vi "InitPneumatic.vi"   [LabVIEW 2015]
uses:
  <vilib>/Rock Robotics/WPI/Utilities/WPI_GetSetVariantRefNum.vi
types:
  T1 = typedef "constants.ctl" = cluster{"motorConstants":cluster{"leftDriveMotor":u8, "rightDriveMotor":u8, "climberAngler":i32, "climberWinch":T2, "shooterTopFlyWheel":T2, "shooterBottomFlyWheel":T2, "climberExtender":i32, "shooterIntakeWheel":T2}, "arduinoInputChannel":cluster{"armAngleUp":i32, "intakeWheelSpinIn":i32, "winchUp":i32, "extenderUp":i32, "AimingAuto":i32, "extenderDown":i32, "FrontArmAxis":i32}, "driveConstants":cluster{"firstIntervalPercent":dbl, "secondIntervalPercent":dbl, "thirdIntervalPercent":dbl}, "cRioInputChanels":cluster{"photoEye":i32, "limitExtender":i32}, "pneumaticsChannels":cluster{"angleSolenoid":T3, "shooterAnglerPneumaticForward":T3, "shooterAnglerPneumaticReverse":T3, "Pneumatics Control Module":u8}, "flyWheelConstants":cluster{"manualTopWheel":dbl, "manualBottomWheel":dbl, "autoFuncConst1":dbl, "autoFuncConst2":dbl, "autoFuncConst3":dbl, "autoFuncConst4":dbl, "Array":dbl[][]}, "Front Arm":cluster{"Arm Motor":u8}}
  T2 = typedef "FPGA_DIOPWMChannel.ctl" = enum8{"PWM 0", "PWM 1", "PWM 2", "PWM 3", "PWM 4", "PWM 5", "PWM 6", "PWM 7", "PWM 8", "PWM 9", "PWM MXP 0", "PWM MXP 1", "PWM MXP 2", "PWM MXP 3", "PWM MXP 4", "PWM MXP 5", "PWM MXP 6", "PWM MXP 7", "PWM MXP 8", "PWM MXP 9", "Invalid"}
  T3 = typedef "WPI_SolenoidChannel.ctl" = enum8{"Solenoid 0", "Solenoid 1", "Solenoid 2", "Solenoid 3", "Solenoid 4", "Solenoid 5", "Solenoid 6", "Solenoid 7", "Invalid"}
  T4 = typedef "WPI_CompressorDevRef.ctl" = cluster{"DevStatus":errorcluster, "Pneumatics Control Module":u8}
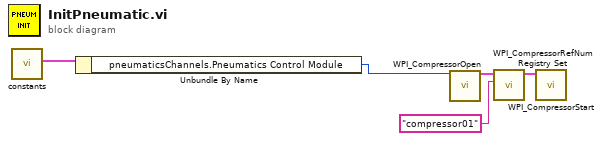
[diagram p0: block diagram]
diagram:
  n1 = call "constants.vi"() -> (2:w2:T1)  [unwired: 11 in]
  n2 = Unbundle By Name(w2) -> ("pneumaticsChannels.Pneumatics Control Module"=w1:u8)
  n3 = call <vilib>:"WPI_CompressorOpen.vi"("Pneumatics Control Module (0)"=w1) -> ("CompressorDevRef"=w3:T4)  [unwired: 13 in, 1 out]
  n4 = call <vilib>:"WPI_CompressorRefNum Registry Set.vi"("refnum name"="compressor01", "CompressorDevRef"=w3) -> ("CompressorDevRef"=w5:T4)  [unwired: 8 in, 1 out]
  n5 = call <vilib>:"WPI_CompressorStart.vi"("CompressorDevRef"=w5) -> ()  [unwired: 9 in, 2 out]
